vi "PiezAlyzer_sub_SaveData.vi"(0 "Array":dbl[][](array[numeric]), 1 "Boolean":bool, 5 "Experiment Name:":string, 7 "File Name:":string, 9 "Cantilever ID:":string, 11 "Sampling frequency:":string, 12 "Actuation Mode:":string) -> ()   [LabVIEW 2013]
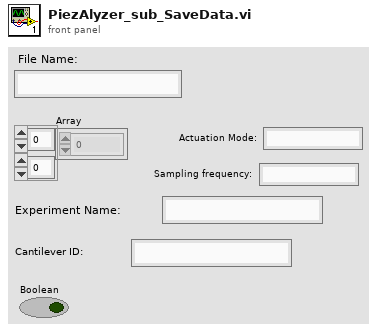
[diagram p1: front panel]
types:
  T1 = enum16{"open", "replace", "create", "open or create", "replace or create", "replace or create with confirmation"}
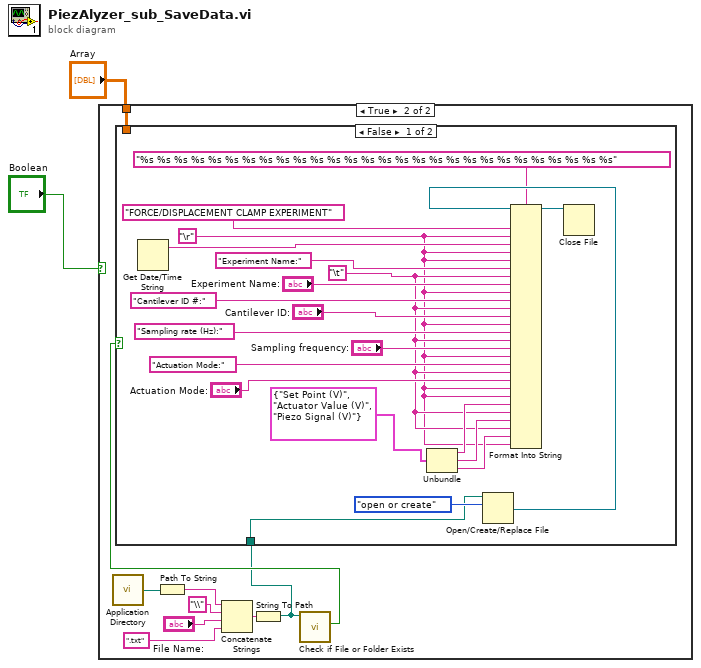
[diagram p0: block diagram]
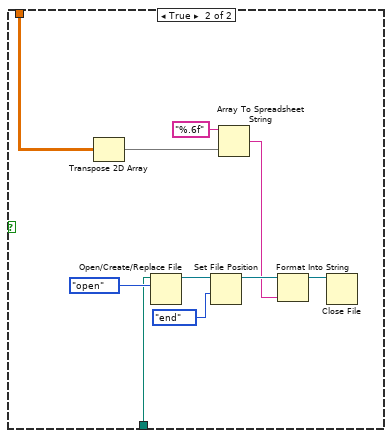
[diagram p3: hidden frame]
diagram:
  n1 = case shown="True" "Boolean" {
    tunnel: "Array" -> [_ w3]
    frame False {
    }
    frame True {
      n2 = call <vilib>:"Application Directory.vi"() -> ("Application Directory"=w9:path)
      n3 = Path To String(path=w9) -> (string=w11:string)
      n4 = Concatenate Strings(w11, "\\", "File Name:", ".txt") -> (w10:string)
      n5 = String To Path(string=w10) -> (path=w4:path)
      n6 = call <vilib>:"Check if File or Folder Exists.vi"("path"=w4) -> ("file or folder exists?"=w5:bool)  [unwired: 8 in, 2 out]
      n7 = case shown="False" w5 {
        tunnel: w4 -> [w18 w41]
        tunnel: w3 -> [_ w34]
        frame False {
          w15 = "\t"
          w13 = "\r"
          n8 = Get Date/Time String() -> (date string=w30:string)  [unwired: 3 in, 1 out]
          n9 = Unbundle(cluster{string, string, string} {"Set Point (V)", "Actuator Value (V)", "Piezo Signal (V)"}) -> (w17:string, w16:string, w14:string)
          n10 = Open/Create/Replace File(file path (use dialog)=w18, operation (0:open)=T1."open or create") -> (refnum out=w28:refnum<file>)  [unwired: 4 in, 2 out]
          n11 = Format Into String ("Format Into File")(format string="%s %s %s %s %s %s %s %s %s %s %s %s %s %s %s %s %s %s %s %s %s %s %s %s %s %s %s %s", initial string=w28, "FORCE/DISPLACEMENT CLAMP EXPERIMENT", w13, w30, w13, w13, "Experiment Name:", w15, "Experiment Name:", w13, "Cantilever ID #:", w15, "Cantilever ID:", w13, "Sampling rate (Hz):", w15, "Sampling frequency:", w13, "Actuation Mode:", w15, "Actuation Mode:", w13, w13, w17, w15, w16, w15, w14, w13) -> (resulting string=w29:refnum<file>)  [unwired: 1 in, 1 out]
          n12 = Close File(refnum=w29) -> ()  [unwired: 1 in, 2 out]
        }
        frame True {
          n13 = Transpose 2D Array(2D array=w34) -> (transposed array=w33:dbl[][])
          n14 = Open/Create/Replace File(file path (use dialog)=w41, operation (0:open)=T1."open") -> (refnum out=w39:refnum<file>)  [unwired: 4 in, 2 out]
          n15 = Set File Position(refnum=w39, from (0:start)=enum16{"start", "end", "current"}."end") -> (refnum out=w37:refnum<file>)  [unwired: 2 in, 1 out]
          n16 = Array To Spreadsheet String(array=w33, 3:"%.6f" ("format string")) -> (spreadsheet string=w36:string)  [unwired: 1 in]
          n17 = Format Into String(initial string=w37, w36) -> (resulting string=w35:refnum<file>)  [unwired: 2 in, 1 out]
          n18 = Close File(refnum=w35) -> ()  [unwired: 1 in, 2 out]
        }
      }
    }
  }
